vi "createdatafile.vi"(8 "error in (no error)":errorcluster, 9 "File Path":path, 10 "Save Video":bool, 11 "Imaging in":refnum<class "Imaging.lvclass">) -> (0 "error out":errorcluster, 3 "Imaging out":refnum<class "Imaging.lvclass">)   [LabVIEW 2014, in "Imaging.lvclass"]
uses:
  Imaging.lvclass
  Imaging.lvclass/Imaging.ctl
  private/HDF5Tools32/LabView/Create Dataset 2D Double.vi
  private/HDF5Tools32/LabView/HDF5Tools.lvlib
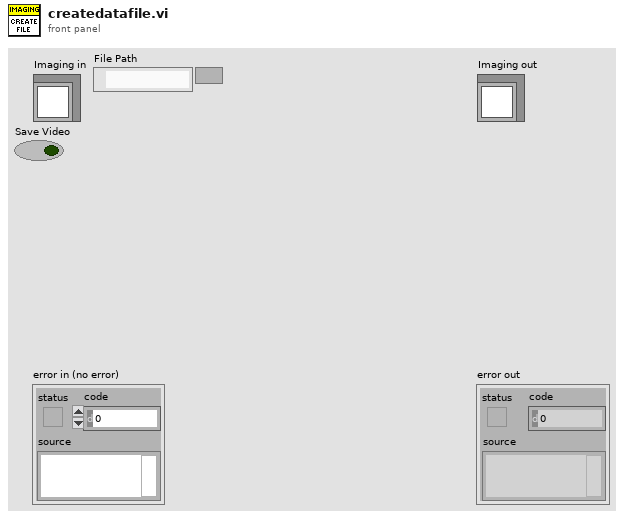
[diagram p1: front panel]
types:
  T1 = typedef "AviRefnum.ctl" = refnum<k1>
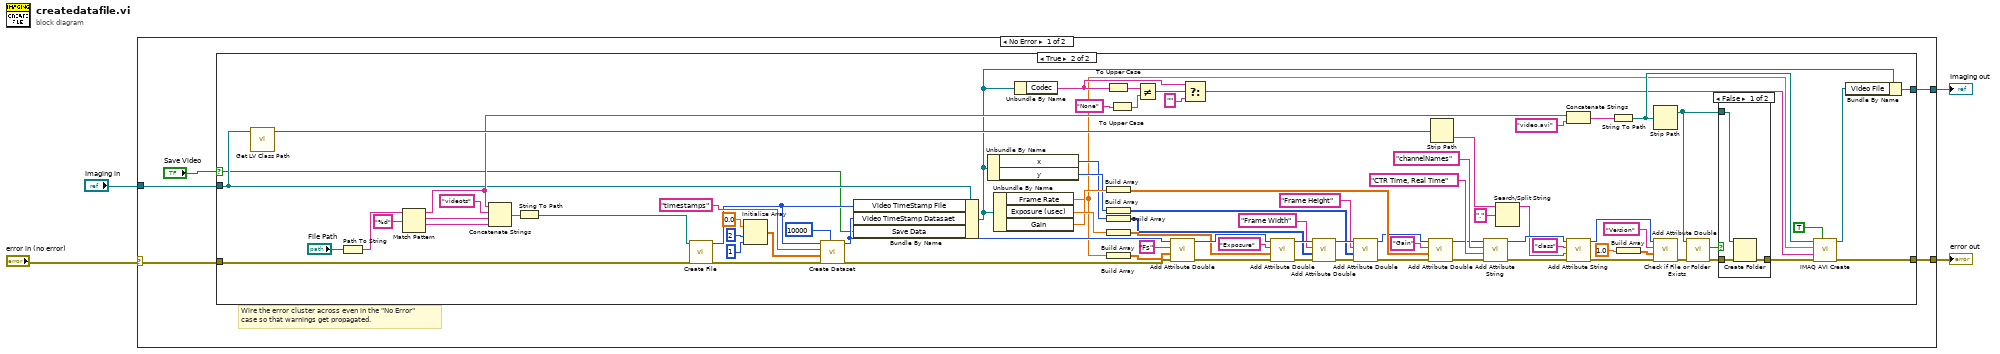
[diagram p0: block diagram]
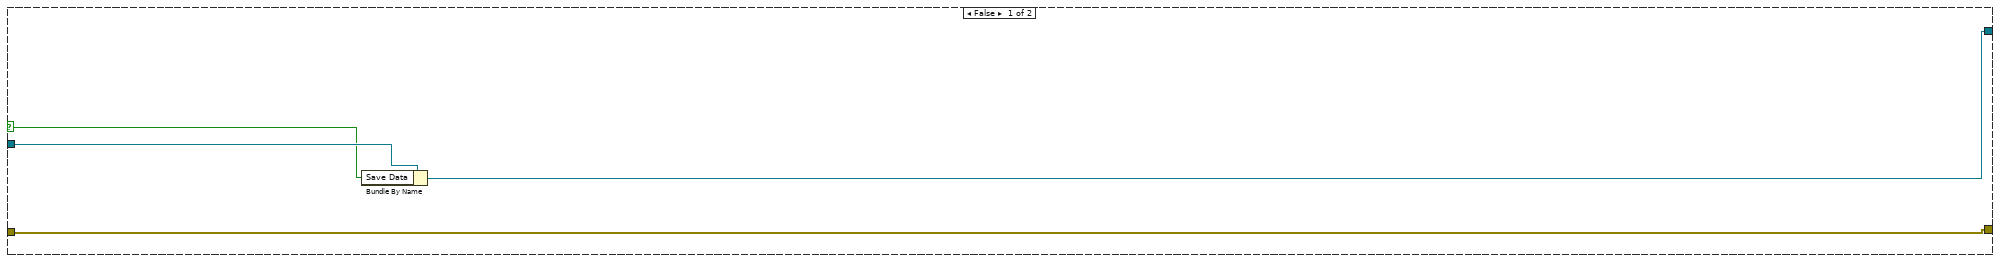
[diagram p2: hidden frame]
diagram:
  n1 = case shown="No Error" "error in (no error)" {
    selector: "error in (no error)" -> [w8 w100]
    tunnel: [w6 w100] -> w3
    tunnel: [w7 w99] -> w1
    tunnel: "Imaging in" -> [w9 w99]
    frame No Error {
      # "Wire the error cluster across even in the \"No Error\"\ncase so that warnings get propagated."
      n2 = case shown="True" "Save Video" {
        selector: "Save Video" -> [w10 w14]
        tunnel: [w11 w30] -> w7
        tunnel: [w13 w28] -> w6
        tunnel: w9 -> [w12 w17]
        tunnel: w8 -> [w13 w15]
        frame False {
          n3 = Bundle By Name(cluster=w12, "Save Data"=w10) -> (w11:refnum<class "Imaging.lvclass">)
        }
        frame True {
          n4 = call <vilib>:"Get LV Class Path.vi"("object"=w17) -> ("class path"=w83:path)  [unwired: 9 in, 1 out]
          n5 = Path To String(path="File Path") -> (string=w70:string)
          n6 = Match Pattern(string=w70, regular expression="%d") -> (before substring=w53:string, match substring=w67:string, after substring=w66:string)  [unwired: 1 in, 1 out]
          n7 = Concatenate Strings(w53, "videots" ("string"), w67, w66) -> (w65:string)
          n8 = String To Path(string=w65) -> (path=w64:path)
          n9 = call "Create File.vi"("Error in"=w15, "File Name"=w64) -> ("Error out"=w94:errorcluster, "file_id"=w44:i32)  [unwired: 6 in]
          n10 = Initialize Array(0.0, 2 ("dimension size"), 1 ("dimension size")) -> (w89:dbl[][])
          n11 = call-poly "Create Dataset.vi"("Chunk size"=10000, "error in (no error)"=w94, "Datatype"=w89, "Dataset name"="timestamps", "Location id in"=w44) -> ("error out"=w85:errorcluster, "Dataset id"=w43:i32)  [unwired: 5 in]
          n12 = Bundle By Name(cluster=w17, "Video TimeStamp File"=w44, "Video TimeStamp Datasaet"=w43, "Save Data"=w14) -> (w27:refnum<class "Imaging.lvclass">)
          n13 = Unbundle By Name(w27) -> ("x"=w33:i32, "y"=w34:i32)
          n14 = Unbundle By Name(w27) -> ("Frame Rate"=w19:dbl, "Exposure (usec)"=w61:dbl, "Gain"=w57:dbl)
          n15 = Unbundle By Name(w27) -> ("Codec"=w22:string)
          n16 = To Upper Case(1:w22) -> (0:w21:string)
          n17 = Build Array(w57) -> (w56:dbl[])
          n18 = Build Array(w34) -> (w31:i32[])
          n19 = Build Array(w33) -> (w32:i32[])
          n20 = Build Array(w61) -> (w60:dbl[])
          n21 = Build Array(w19) -> (w87:dbl[])
          n22 = To Upper Case(1:"None" ("y")) -> (0:w24:string)
          n23 = Not Equal?(x=w21, y=w24) -> (x != y?=w25:bool)
          n24 = call "Add Attribute Double.vi"("error in (no error)"=w85, "data"=w87, "Attribute name"="Fs", "loc_id"=w43) -> ("error out"=w59:errorcluster, "loc_id_out"=w63:i32)  [unwired: 6 in]
          n25 = Select(t=w22, s=w25, f="") -> (s? t:f=w26:string)
          n26 = call "Add Attribute Double.vi"("error in (no error)"=w59, "data"=w60, "Attribute name"="Exposure", "loc_id"=w63) -> ("error out"=w40:errorcluster, "loc_id_out"=w42:i32)  [unwired: 6 in]
          n27 = call "Add Attribute Double.vi"("error in (no error)"=w40, "data"=w32, "Attribute name"="Frame Width", "loc_id"=w42) -> ("error out"=w39:errorcluster, "loc_id_out"=w41:i32)  [unwired: 6 in]
          n28 = call "Add Attribute Double.vi"("error in (no error)"=w39, "data"=w31, "Attribute name"="Frame Height", "loc_id"=w41) -> ("error out"=w36:errorcluster, "loc_id_out"=w35:i32)  [unwired: 6 in]
          n29 = call "Add Attribute Double.vi"("error in (no error)"=w36, "data"=w56, "Attribute name"="Gain", "loc_id"=w35) -> ("error out"=w54:errorcluster, "loc_id_out"=w55:i32)  [unwired: 6 in]
          n30 = Strip Path(path=w83) -> (name=w82:string)  [unwired: 1 out]
          n31 = call "Add Attribute String.vi"("error in (no error)"=w54, "Attribute data"="CTR Time, Real Time", "Attribute name"="channelNames", "loc_id"=w55) -> ("error out"=w79:errorcluster, "loc_id_out"=w84:i32)  [unwired: 6 in]
          n32 = Search/Split String(string=w82, search string/char (-)=".") -> (substring before match=w78:string)  [unwired: 1 in, 2 out]
          n33 = Concatenate Strings(w53, "video.avi" ("string")) -> (w51:string)
          n34 = call "Add Attribute String.vi"("error in (no error)"=w79, "Attribute data"=w78, "Attribute name"="class", "loc_id"=w84) -> ("error out"=w75:errorcluster, "loc_id_out"=w73:i32)  [unwired: 6 in]
          n35 = String To Path(string=w51) -> (path=w45:path)
          n36 = Build Array(1.0) -> (w74:dbl[])
          n37 = Strip Path(path=w45) -> (stripped path=w49:path)  [unwired: 1 out]
          n38 = call "Add Attribute Double.vi"("error in (no error)"=w75, "data"=w74, "Attribute name"="Version", "loc_id"=w73) -> ("error out"=w48:errorcluster)  [unwired: 6 in, 1 out]
          n39 = call <vilib>:"Check if File or Folder Exists.vi"("error in (no error)"=w48, "path"=w49) -> ("error out"=w47:errorcluster, "file or folder exists?"=w50:bool)  [unwired: 7 in, 1 out]
          n40 = case shown="False" w50 {
            tunnel: w49 -> [w97 _]
            tunnel: w47 -> [w96 w98]
            tunnel: [w95 w98] -> w46
            frame False {
              n41 = Create Folder(path (use dialog)=w97, error in=w96) -> (error out=w95:errorcluster)  [unwired: 1 in, 2 out]
            }
            frame True {
            }
          }
          n42 = call "IMAQ AVI Create"("Has Data"=TRUE, "error in (no error)"=w46, "Compression Filter"=w26, "Frames Per Second"=w19, "AVI Path"=w45) -> ("error out"=w28:errorcluster, "Avi Refnum"=w29:T1)  [unwired: 2 in, 3 out]
          n43 = Bundle By Name(cluster=w27, "Video File"=w29) -> (w30:refnum<class "Imaging.lvclass">)
        }
      }
    }
    frame Error {
    }
  }
  "error out" <- w3
  "Imaging out" <- w1
